vi "TestMotor.vi"() -> ()   [LabVIEW 2017]
panel:
  in  "Motor 1 Encoder Target":i32(slide) scale=-100.0..100.0
  in  "Motor 2 Encoder Target":i32(slide) scale=-100.0..100.0
  in  "Motor 1 Contant Speed (Degrees per Second)":i16(slide) scale=-100.0..100.0
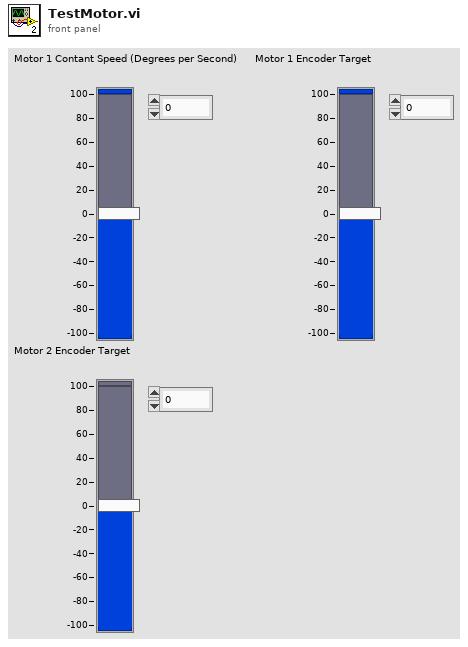
[diagram p1: front panel]
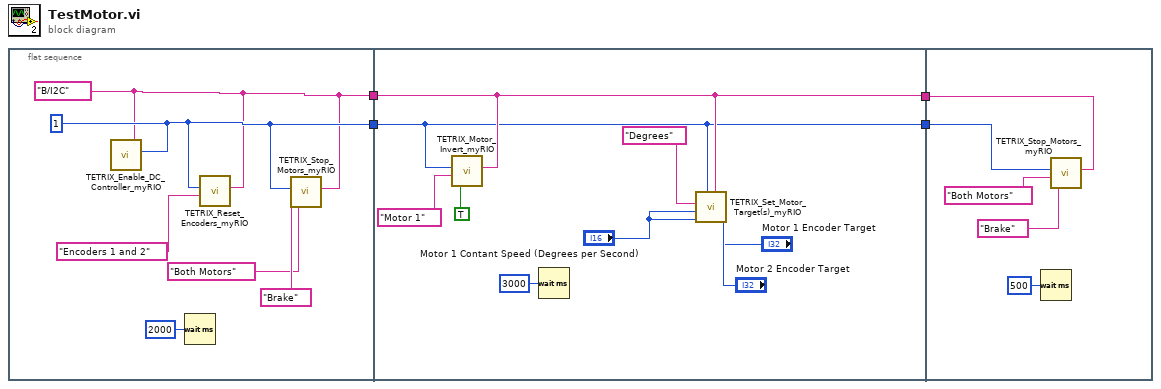
[diagram p0: block diagram]
diagram:
  n1 = flat-sequence {
    tunnel: [w6] -> w4
    tunnel: [w5] -> w3
    tunnel: w4 -> [w11]
    tunnel: w3 -> [w12]
    tunnel: [w11] -> w2
    tunnel: [w12] -> w1
    tunnel: w2 -> [w22]
    tunnel: w1 -> [w21]
    frame #0 {
      w5 = tag "B/I2C" ("myRIO MXP Port A/B")
      w6 = u8 1 ("Controller ID#  (I2C Address)")
      n2 = call <vilib>:"TETRIX_Enable_DC_Controller_myRIO.vi"("myRIO MXP Port A/B"=w5, "Controller ID#  (I2C Address)"=w6) -> ()  [unwired: 5 in, 1 out]
      n3 = Wait (ms)(milliseconds to wait=u32 2000) -> ()  [unwired: 1 out]
      n4 = call <vilib>:"TETRIX_Reset_Encoders_myRIO.vi"("myRIO MXP Port A/B"=w5, "Select Encoder"="Encoders 1 and 2", "Controller ID#  (I2C Address)"=w6) -> ()  [unwired: 4 in, 1 out]
      n5 = call <vilib>:"TETRIX_Stop_Motors_myRIO.vi"("myRIO MXP Port A/B"=w5, "Stop Mode"="Brake", "Select Channel"="Both Motors", "Controller ID#  (I2C Address)"=w6) -> ()  [unwired: 3 in, 1 out]
    }
    frame #1 {
      n6 = call <vilib>:"TETRIX_Motor_Invert_myRIO.vi"("myRIO MXP Port A/B"=w12, "Invert State"=TRUE, "Select Channel"="Motor 1", "Controller ID#  (I2C Address)"=w11) -> ()  [unwired: 3 in, 1 out]
      n7 = Wait (ms)(milliseconds to wait=u32 3000) -> ()  [unwired: 1 out]
      n8 = call <vilib>:"TETRIX_Set_Motor_Target(s)_myRIO.vi"("Motor 2 Encoder Target"="Motor 2 Encoder Target", "Motor 1 Encoder Target"="Motor 1 Encoder Target", "myRIO MXP Port A/B"=w12, "Controller ID#  (I2C Address)"=w11, "Motor 2 Constant Speed (Degrees per Second)"="Motor 1 Contant Speed (Degrees per Second)", "Motor 1 Contant Speed (Degrees per Second)"="Motor 1 Contant Speed (Degrees per Second)", "Encoder Units"="Degrees") -> ()  [unwired: 2 in, 1 out]
    }
    frame #2 {
      n9 = Wait (ms)(milliseconds to wait=u32 500) -> ()  [unwired: 1 out]
      n10 = call <vilib>:"TETRIX_Stop_Motors_myRIO.vi"("myRIO MXP Port A/B"=w21, "Stop Mode"="Brake", "Select Channel"="Both Motors", "Controller ID#  (I2C Address)"=w22) -> ()  [unwired: 3 in, 1 out]
    }
  }
